vi "Gas_Density.vi"(1 "Pressure (mbar)":dbl=1000.0 format="%.2f", 2 "Temperature (C)":dbl format="%.2f", 3 "Gas":T1="Air") -> (0 "Density (kg/m^3) (= g/l)":dbl=nan format="%_6f")   [LabVIEW 2021]
uses:
  Anemometry/Anemometry Sub Vis/Controls/GasCombo.ctl
panel:
  out "rhoVdW":dbl
  out "rhoIdeal":dbl
  out "VdWvol(l)":dbl
  out "idealVol(l)":dbl
  out "diff%":dbl format="%#_3f"
  in  "uncorrected":bool
  out "MW (g/mol) (=kg/kmol)":dbl
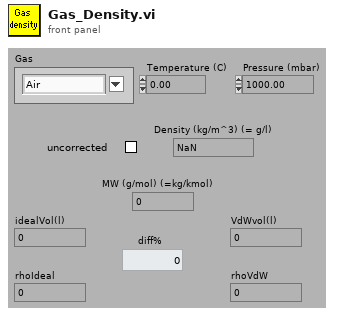
[diagram p1: front panel]
types:
  T1 = typedef "GasCombo.ctl" = string
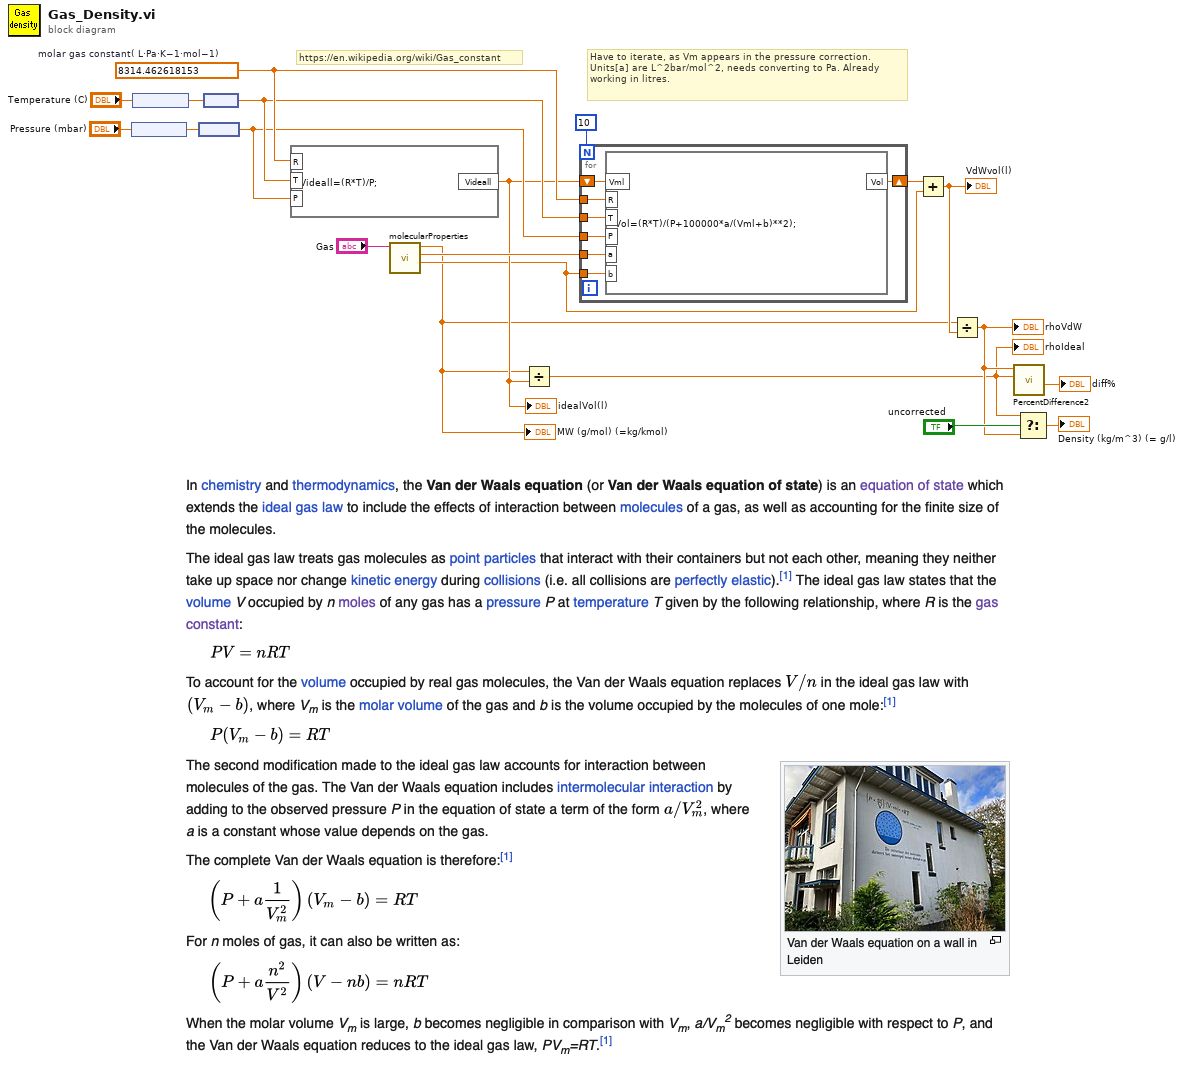
[diagram p0: block diagram]
diagram:
  w10 = 8314.462618153  # molar gas constant(	L⋅Pa⋅K−1⋅mol−1)
  # "https://en.wikipedia.org/wiki/Gas_constant"
  # "Have to iterate, as Vm appears in the pressure correction.\nUnits[a] are L^2bar/mol^2, needs converting to Pa. Already working in litres."
  n1 = node("Pressure (mbar)") -> (w13:dbl[unit])
  n2 = node("Temperature (C)") -> (w15:dbl[unit])
  n3 = node(w13) -> (w8:dbl)
  n4 = node(w15) -> (w9:dbl)
  n5 = formula code="Videall=(R*T)/P;"("R"=w10, "T"=w9, "P"=w8) -> ("Videall"=w5:dbl)
  "idealVol(l)" <- w5
  n6 = call "molecularProperties.vi"("Gas"="Gas") -> ("VdWb(L/mol)"=w2:dbl, "VdWa(L^2bar/mol^2)"=w11:dbl, "Molecular Weight"=w1:dbl)  [unwired: 8 in]
  "MW (g/mol) (=kg/kmol)" <- w1
  n7 = Divide(x=w1, y=w5) -> (x/y=w3:dbl)
  "rhoIdeal" <- w3
  n8 = for {
    N: 10 -> [_]
    shift-right: [w21] -> w7
    shift-left: w5 -> [w27]
    tunnel: w9 -> [w25]
    tunnel: w10 -> [w26]
    tunnel: w8 -> [w24]
    tunnel: w11 -> [w23]
    tunnel: w2 -> [w22]
    n9 = formula code="Vol=(R*T)/(P+100000*a/(Vml+b)**2);"("Vml"=w27, "R"=w26, "T"=w25, "P"=w24, "a"=w23, "b"=w22) -> ("Vol"=w21:dbl)
  }
  n10 = Add(x=w7, y=w2) -> (x+y=w6:dbl)
  "VdWvol(l)" <- w6
  n11 = Divide(x=w1, y=w6) -> (x/y=w4:dbl)
  "rhoVdW" <- w4
  n12 = call "PercentDifference2.vi"("target"=w3, "achieved"=w4) -> ("error%"=→"diff%":dbl)  [unwired: 8 in, 1 out]
  n13 = Select(t=w3, s="uncorrected", f=w4) -> (s? t:f=→"Density (kg/m^3) (= g/l)":dbl)
